vi "Read Current Measurement.vi"   [LabVIEW 2013, in "Cal Inst.lvlib" / "California Instruments iX Series.lvlib"]
doc: "Reads single or multiple current measurement(s)."
uses:
  California Instruments iX Series.lvlib
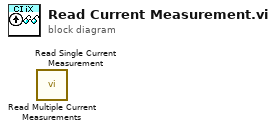
[diagram p0: block diagram]
diagram:
  n1 = call "Read Multiple Current Measurements.vi"() -> ()  [unwired: 9 in, 3 out]
  n2 = call "Read Single Current Measurement.vi"() -> ()  [unwired: 9 in, 3 out]
